vi "Configure Trigger Hold.vi"(0 "VISA resource name":refnum<visa-resource-name>, 5 "Enable Trigger Hold (F:Disable)":bool, 7 "Hold Time (0.0001s)":dbl=0.0001 min=0.0 max=1.0 format="%.6f", 11 "error in (no error)":errorcluster) -> (4 "VISA resource name out":refnum<visa-resource-name>, 15 "error out":errorcluster)   [LabVIEW 2020, in "Anritsu Signal Analyzer Series.lvlib"]
doc: "Configures the trigger hold settings of the spectrum analyzer."
uses:
  Anritsu Signal Analyzer Series.lvlib
panel:
  # "s"
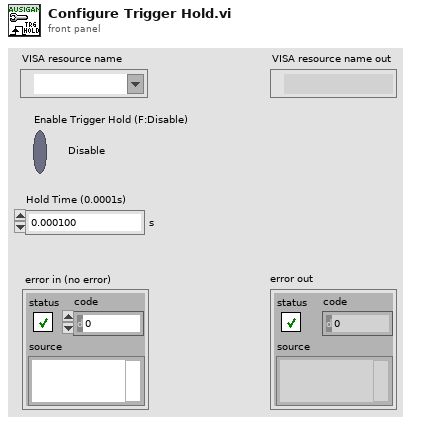
[diagram p1: front panel]
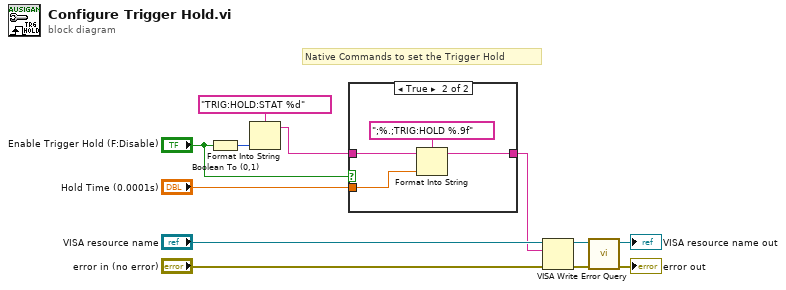
[diagram p0: block diagram]
diagram:
  # "Native Commands to set the Trigger Hold"
  n1 = Boolean To (0,1)(Boolean="Enable Trigger Hold (F:Disable)") -> (0, 1=w4:i16)
  n2 = Format Into String(format string="TRIG:HOLD:STAT %d" ("_CommandSet"), w4) -> (resulting string=w3:string)  [unwired: 2 in, 1 out]
  n3 = case shown="True" "Enable Trigger Hold (F:Disable)" {
    tunnel: "Hold Time (0.0001s)" -> [_ w17]
    tunnel: w3 -> [w13 w15]
    tunnel: [w13 w14] -> w1
    frame False {
    }
    frame True {
      n4 = Format Into String(format string=";%.;TRIG:HOLD %.9f" ("Format String"), initial string=w15, w17) -> (resulting string=w14:string)  [unwired: 1 in, 1 out]
    }
  }
  n5 = VISA Write(VISA resource name="VISA resource name", write buffer=w1, error in (no error)="error in (no error)") -> (VISA resource name out=w6:refnum<visa-resource-name>, error out=w7:errorcluster)  [unwired: 1 out]
  n6 = call "Error Query.vi"("error in (no error)"=w7, "VISA resource name"=w6) -> ("error out"=→"error out":errorcluster, "VISA resource name out"=→"VISA resource name out":refnum<visa-resource-name>)  [unwired: 6 in, 2 out]
